vi "event_smartconfig_processing.vi"(11 "message":string) -> ()   [LabVIEW 2014]
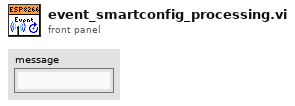
[diagram p1: front panel]
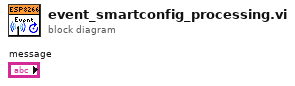
[diagram p0: block diagram]
diagram:
